vi "midi_in.connect.vi"(8 "error in (no error)":errorcluster, 10 "device_index":i32, 11 "LabVIEW-MIDI-XPLAT in":refnum<class "LabVIEW-MIDI-XPLAT.lvclass">) -> (0 "error out":errorcluster, 2 "Return":i32, 3 "LabVIEW-MIDI-XPLAT out":refnum<class "LabVIEW-MIDI-XPLAT.lvclass">)   [LabVIEW 2020, in "LabVIEW-MIDI-XPLAT.lvclass"]
uses:
  LabVIEW-MIDI-XPLAT.lvclass
  LabVIEW-MIDI-XPLAT.lvclass/LabVIEW-MIDI-XPLAT.ctl
  target/release/midi_driver.dll
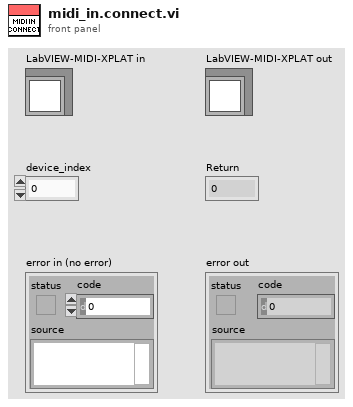
[diagram p1: front panel]
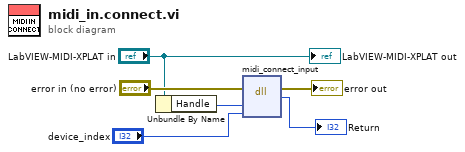
[diagram p0: block diagram]
diagram:
  n1 = Unbundle By Name("LabVIEW-MIDI-XPLAT in") -> ("Handle"=w3:i32)
  n2 = dll-call lib="C:/code/LabVIEW-MIDI-XPLAT/target/release/midi_driver.dll" fn="midi_connect_input"(error in="error in (no error)", "handle"=w3, "device_index"="device_index") -> (error out=→"error out":errorcluster, "Return"=→"Return":i32)  [unwired: 4 in, 1 out]
  "LabVIEW-MIDI-XPLAT out" <- "LabVIEW-MIDI-XPLAT in"
